vi "PH_Beamline.Calc Mirrortower State.vi"(0 "i ref in":refnum<vi>, 2 "PA Exit closed or shining into LL":bool, 3 "Not shining to Mirrortower":bool, 5 "error in (no error)":errorcluster) -> (14 "i ref out":refnum<vi>, 19 "error out":errorcluster)   [LabVIEW 2014, in "PH_Beamline.lvlib"]
doc: "This VI calculates the Mirrortower state of the Beamline."
uses:
  PH_Beamline.lvlib
  PH_StatusHandler/PH_StatusHandler.Status.ctl
  PH_StatusHandler/PH_StatusHandler.lvlib
  PH_Common/PH_Common.lvlib
  PH_BL-Master/PH_BL-Master.lvlib
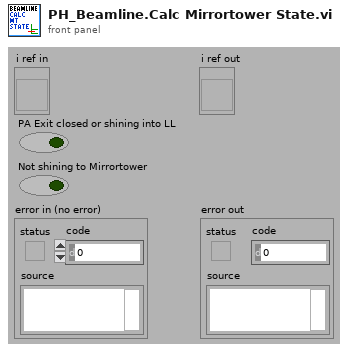
[diagram p1: front panel]
types:
  T1 = typedef "PH_Beamline.lvlib/PH_Beamline.i attribute.ctl" = cluster{"GUI Refs":cluster{"PA ok":refnum<vi>, "MA ok":refnum<vi>, "fs FE ok":refnum<vi>, "ns FE ok":refnum<vi>, "PA ED ok":refnum<vi>, "MAS ok":refnum<vi>, "Booster ok":refnum<vi>, "Mirrortower ok":refnum<vi>, "In.-Box ok":refnum<vi>, "Compressor ok":refnum<vi>, "Experiment LB ok":refnum<vi>, "Experiment LL ok":refnum<vi>, "PHELIX_Beckhoff_Watchdog":refnum<vi>, "Shutters closed":refnum<vi>, "uOPA ok":refnum<vi>, "Vacuum no shotcond Comp LB":refnum<vi>}, "Refs BL MA":refnum<vi>[], "Refs BL MA-IB":refnum<vi>[], "Refs BL fs":refnum<vi>[], "Refs BL PA ED":refnum<vi>[], "Refs BL MAS":refnum<vi>[], "Refs BL Boo":refnum<vi>[], "Refs BL ns":refnum<vi>[], "Refs BL Mirrortower":refnum<vi>[], "Refs BL Compressor":refnum<vi>[], "Refs BL Exp LB":refnum<vi>[], "Radiation Safety":cluster{"Exp Laserbay":cluster{"Ref Op Mode":refnum<vi>, "Ref Laserbay evacuated":refnum<vi>, "Tagname LB evacuated":string, "Shot Mode":T2, "Laserbay evacuated?":i32, "Tagname HV room locked":string, "HV room locked?":i32, "Ref HV room locked":refnum<vi>, "Tagname bridged?":string, "Ref Bridge":refnum<vi>, "I<1E18W/cm²":bool}, "Exp Laserlab":cluster{"Ref Op Mode":refnum<vi>, "Ref Laserlab evacuated":refnum<vi>, "Tagname LL evacuated":string, "Shot Mode":T2, "Laserlab evacuated?":i32, "Tagname bridged?":string, "Ref Bridge":refnum<vi>, "I<1E18W/cm²":bool}}, "Refs BL LL":refnum<vi>[], "PP Igni Heating GUI Refs":refnum<vi>[], "PP Igni Heating Tagnames ":string[], "Refs BL PA":cluster{"undelayed Line before Shutter":refnum<vi>[], "undelayed Line after Shutter":refnum<vi>[], "before Bypass":refnum<vi>[], "delayed Line before Shutter":refnum<vi>[], "delayed Line after Shutter":refnum<vi>[], "before Shutter Input":refnum<vi>[], "after Shutter Input":refnum<vi>[], "Bypass":refnum<vi>[], "before Shutter Exit":refnum<vi>[], "after Shutter Exit":refnum<vi>[], "to MA":refnum<vi>[], "to Lab":refnum<vi>[]}, "BL":cluster{"YLF_BL_Status":i32, "fs_BL_Status":i32, "fs_YLF_BL_Status":i32, "ns_BL_Status":i32, "PA_Input_BL_Status":i32, "PA_UnDelay_BL_Status":i32, "PA_Delay_BL_Status":i32, "PA_BL_Status":i32, "PA_Bypass_BL_Status":i32, "PA_Exit_BL_Status":i32, "PA_LL_BL_Status":i32, "LL_BL_Status":i32, "PA_MA_BL_Status":i32, "MA_Exit_BL_Status":i32, "MA_Z6_BL_Status":i32, "Z6_BL_Status":i32, "MA_LB_BL_Status":i32, "LB_TB2_BL_Status":i32, "PA_before_Bypass_BL_Status":i32, "LB_TB3_BL_Status":i32}, "State Subsystems":cluster{"PA":bool, "MA":bool, "ns FE":bool, "fs FE":bool, "PA ED":bool, "In.-Box":bool, "MAS":bool, "Booster":bool, "Mirrortower":bool, "Compressor":bool, "Experiment LB":bool, "Experiment LL":bool, "uOPA":bool}, "Status Subscriber Information":T3, "Refs BL uOPA":refnum<vi>[], "PA_Input_2_Beam_6PWpGUI not linked?":bool, "PA_Input_Delay_6PGUI not linked?":bool, "Settings":T6}
  T2 = typedef "PH_Beamline.lvlib/PH_Beamline.Operation Mode.ctl" = i32
  T3 = typedef "PH_Beamline.lvlib/PH_Beamline.Status Subscriber Information.ctl" = cluster{"fs Swich YLF":T4, "fs Exit Shutter":T4, "ns Exit Shutter":T4, "PA Input Shutter":T4, "PA PC WP":T4, "PA PC WP 2":T4, "PA Bypass In":T4, "PA Bypass Out":T4, "PA CH 1":T4, "PA delayed":T4, "PA non delayed":T4, "PA Exit Shutter":T4, "PA Switch Lab":T4, "PA Bridge CH Input MA":T4, "MA Diffusor IB":T4, "MA IB Ready":T4, "MA CH 1":T4, "MA CH 2":T4, "MA CH 3":T4, "MA CH 4":T4, "MA Shutter Align Cam":T4, "MA Position MM5":T4, "Calorimeter Switch":T4, "BL Z6 CH 9":T4, "BL Z6 Beamdump":T4, "BL Z6 Shutter":T4, "COS Sensitivity Switch":T4, "Exp LB Shutter":T4, "Exp LB TB 2":T4, "Exp LB TB 3":T4, "PA LL Input CH":T4, "PA LL Output CH":T4, "LL Comp Input Shutter":T4, "LL Comp Output Shutter":T4, "LL Comp FF Shutter":T4, "Exp LL Shutter":T4, "MA IM In IB":T4, "MA IM Out IB":T4, "MA DB In IB":T4, "MA DB Out IB":T4, "Exp LB Shutter Interlock":T4, "Exp LL Shutter Interlock":T4, "MM1 Force Sensor":T4}
  T4 = typedef "PH_BL-Master.lvlib/PH_BL-Master.Status Subscriber Information.ctl" = cluster{"Index of element":i32, "Attributeset":T5}
  T5 = typedef "PH_BL-Master.lvlib/PH_BL-Master.Attribute Set.ctl" = enum16{"Boolean Status Service Subscriber", "Picture Status Service Subscriber"}
  T6 = typedef "PH_Beamline_Chief.lvlib/PH_Beamline_Chief.Settings.ctl" = cluster{"PA Doublepass Mode":bool, "Compressor Vaccuum LB not relevant":bool, "Windowshutter TB2 not relevant":bool, "Windowshutter TB3 not relevant":bool}
  T7 = enum16{"All, Default", "PreAmp", "MainAmp", "Compressor", "Experiment", "Z6 Telescope"}
  T8 = typedef "PH_StatusHandler.lvlib/PH_StatusHandler.Status.ctl" = i16
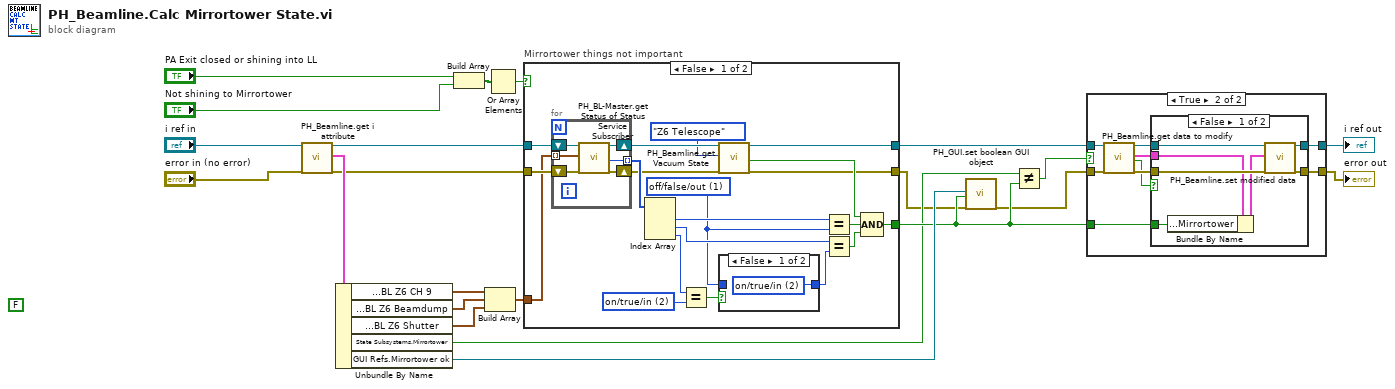
[diagram p0: block diagram]
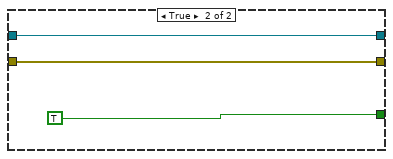
[diagram p5: hidden frame]
diagram:
  (unwired) FALSE ("Not shining to Mirrortower")
  n1 = call "PH_Beamline.get i attribute.vi"("i ref in"="i ref in", "error in (no error)"="error in (no error)") -> ("i ref out"=w3:refnum<vi>, "i attribute"=w12:T1, "error out"=w2:errorcluster)  [unwired: 15 in]
  n2 = Unbundle By Name(w12) -> ("Status Subscriber Information.BL Z6 CH 9"=w8:T4, "Status Subscriber Information.BL Z6 Beamdump"=w7:T4, "Status Subscriber Information.BL Z6 Shutter"=w9:T4, "State Subsystems.Mirrortower"=w17:bool, "GUI Refs.Mirrortower ok"=w21:refnum<vi>)
  n3 = Build Array("PA Exit closed or shining into LL", "Not shining to Mirrortower") -> (w20:bool[])
  n4 = Build Array(w8, w7, w9) -> (w6:T4[])
  n5 = Or Array Elements(Boolean array=w20) -> (logical OR=w22:bool)
  n6 = case "Mirrortower things not important" shown="False" w22 {
    tunnel: w3 -> [w31 w53]
    tunnel: [w25 w53] -> w11
    tunnel: w2 -> [w32 w52]
    tunnel: [w24 w52] -> w10
    tunnel: [w41 TRUE] -> w18
    tunnel: w6 -> [w29 _]
    frame False {
      w34 = T8 1 items=["no info", "off/false/out", "on/true/in", "Failure", "Alarm", "Status 1", "Status 2", "Status 3"] ("x")
      w38 = T8 2 items=["no info", "off/false/out", "on/true/in", "Failure", "Alarm", "Status 1", "Status 2", "Status 3"] ("y")
      n7 = for {
        tunnel: [w46] -> w39 mode=indexing
        tunnel: w29 -> [w45] mode=indexing
        shift-right: [w49] -> w26
        shift-left: w31 -> [w50]
        shift-right: [w47] -> w27
        shift-left: w32 -> [w48]
        n8 = call "PH_BL-Master.get Status of Status Service Subscriber.vi"("i ref in"=w50, "Wanted Status Subscriber Information"=w45, "error in (no error)"=w48) -> ("i ref out"=w49:refnum<vi>, "Status"=w46:T8, "error out"=w47:errorcluster)  [unwired: 11 in, 3 out]
      }
      n9 = Index Array(array=w39) -> (element #1=w40:T8, element #2=w36:T8, element #3=w30:T8)  [unwired: 3 in]
      n10 = Equal?(x=w30, y=w38) -> (x = y?=w37:bool)
      n11 = call "PH_Beamline.get Vacuum State.vi"("i ref in"=w26, "Subsystem"=T7."Z6 Telescope", "error in (no error)"=w27) -> ("i ref out"=w25:refnum<vi>, "vacua in range"=w28:bool, "error out"=w24:errorcluster)  [unwired: 14 in]
      n12 = case shown="False" w37 {
        tunnel: w34 -> [_ w44]
        tunnel: [w43 w44] -> w33
        frame False {
          w43 = T8 2 items=["no info", "off/false/out", "on/true/in", "Failure", "Alarm", "Status 1", "Status 2", "Status 3"] ("x")
        }
        frame True {
        }
      }
      n13 = Equal?(x=w40, y=w34) -> (x = y?=w42:bool)
      n14 = Equal?(x=w36, y=w33) -> (x = y?=w35:bool)
      n15 = Compound Arithmetic op=AND(w28, w42, w35) -> (w41:bool)
    }
    frame True {
    }
  }
  n16 = call "PH_GUI.set boolean GUI object.vi"("Boolean Knob GUI Ref"=w21, "Value"=w18, "error in (no error)"=w10) -> ("error out"=w16:errorcluster)  [unwired: 16 in]
  n17 = Not Equal?(x=w17, y=w18) -> (x != y?=w19:bool)
  n18 = case shown="True" w19 {
    tunnel: [w55 w60] -> w14
    tunnel: [w54 w59] -> w15
    tunnel: w18 -> [_ w58]
    tunnel: w16 -> [w54 w57]
    tunnel: w11 -> [w55 w56]
    frame False {
    }
    frame True {
      n19 = call "PH_Beamline.get data to modify.vi"("i ref in"=w56, "error in (no error)"=w57) -> ("i ref out"=w63:refnum<vi>, "i attribute"=w61:T1, "timed out"=w62:bool, "error out"=w64:errorcluster)  [unwired: 14 in]
      n20 = case shown="False" w62 {
        tunnel: w64 -> [w71 w72]
        tunnel: w63 -> [w70 w73]
        tunnel: [w69 w72] -> w59
        tunnel: [w68 w73] -> w60
        tunnel: w61 -> [w67 _]
        tunnel: w58 -> [w65 _]
        frame False {
          n21 = Bundle By Name(cluster=w67, "State Subsystems.Mirrortower"=w65) -> (w66:T1)
          n22 = call "PH_Beamline.set modified data.vi"("i ref in"=w70, "i attribute"=w66, "error in (no error)"=w71) -> ("i ref out"=w68:refnum<vi>, "error out"=w69:errorcluster)  [unwired: 15 in]
        }
        frame True {
        }
      }
    }
  }
  "i ref out" <- w14
  "error out" <- w15
